vi "cic4_test.vi"() -> ()   [LabVIEW 2013]
uses:
  <vilib>/rvi/FXPMathLib/FxpConvert/subVIs/nifxpmath_Convert_SimConfig.ctl
  <vilib>/fxp/LVFixedPointQuantizationPolicyTypeDef.ctl
  <vilib>/fxp/LVFixedPointOverflowPolicyTypeDef.ctl
  <vilib>/rvi/FXPMathLib/FxpConvert/simVIs/DllFxpConvertTemp_sub.vi
  <vilib>/rvi/FXPMathLib/FxpInterpret/XNode/nifxpmath_Interpret.xnode
  <vilib>/rvi/FXPMathLib/FxpConvert/XNode/nifxpmath_Convert.xnode
panel:
  out "rdy fro data":bool[](array[boolean])
  out "Array 4":fxp<+/-,25,19>[](array[numeric])
  out "Array 3":bool[](array[boolean])
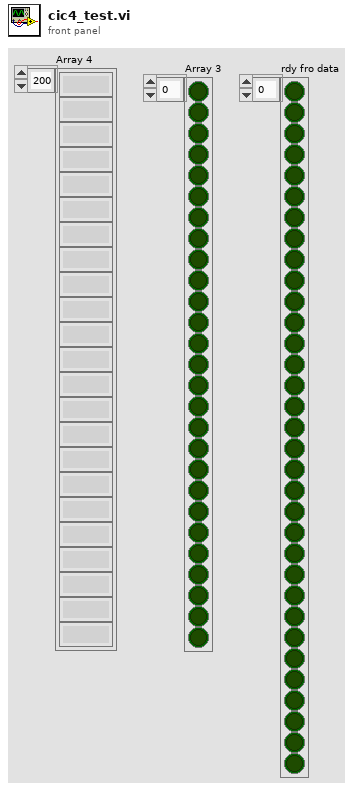
[diagram p1: front panel]
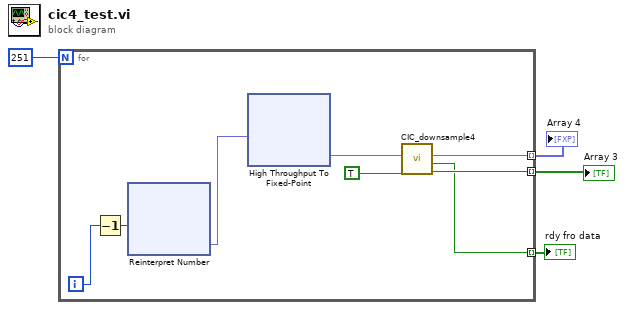
[diagram p0: block diagram]
diagram:
  n1 = for {
    N: 251 -> [_]
    tunnel: [w8] -> w3 mode=indexing
    tunnel: [w7] -> w2 mode=indexing
    tunnel: [w5] -> w1 mode=indexing
    i -> [w12]
    n2 = Decrement(x=w12) -> (x-1=w10:i32)
    n3 = xnode "Reinterpret Number"("x"=w10) -> ("y"=w11:fxp<+/-,32,32>)
    n4 = xnode "High Throughput To Fixed-Point"("x"=w11) -> ("y"=w9:fxp<+/-,20,16>)
    n5 = call "CIC_downsample4.vi"("valid in"=TRUE, "din"=w9) -> ("valid out"=w7:bool, "rdy for data"=w5:bool, "dout"=w8:fxp<+/-,25,19>)  [unwired: 7 in]
  }
  "Array 3" <- w2
  "Array 4" <- w3
  "rdy fro data" <- w1
